vi "Data operation.vi"(8 "Output list":dbl[](array[numeric]), 9 "Operation":enum16{"Increase", "maintain", "Decrease"}(ring), 10 "Keithley Output Configure":T1={"Sample Count (10)"=10, "Timeout (10000 ms)"=10000, "Compliance  Level (0.1)"=0.1, "Output Level (0)"=0.0, "Source Mode  (0: Voltage)"=0, "Output sequence"=0, "Output list"=[]} {"Source Mode  (0: Voltage)" items=["Voltage", "Current"]; "Timeout (10000 ms)" format="%#.6g"}) -> (2 "Keithley Output Configure 2":T1={"Sample Count (10)"=10, "Timeout (10000 ms)"=10000, "Compliance  Level (0.1)"=0.1, "Output Level (0)"=0.0, "Source Mode  (0: Voltage)"=0, "Output sequence"=0, "Output list"=[]} {"Source Mode  (0: Voltage)" items=["Voltage", "Current"]; "Timeout (10000 ms)" format="%#.6g"})   [LabVIEW 2017]
uses:
  controls/Keithley input.ctl
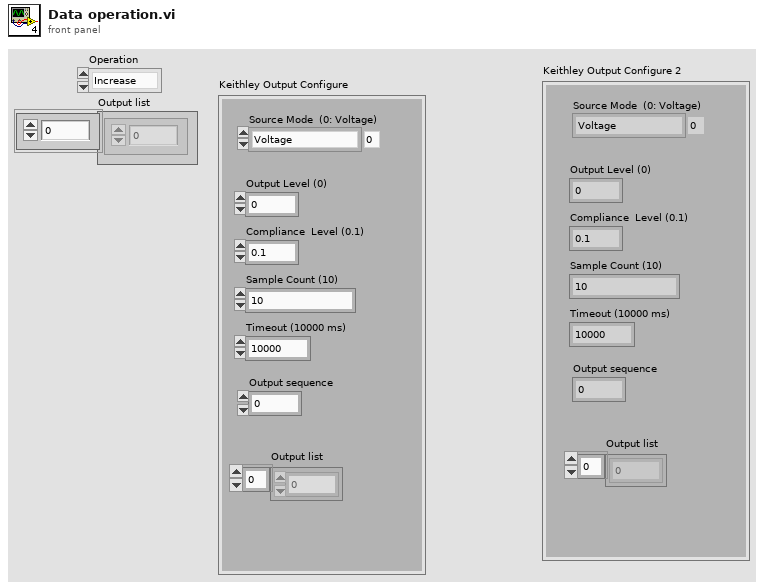
[diagram p1: front panel]
types:
  T1 = typedef "Keithley input.ctl" = cluster{"Sample Count (10)":i32, "Timeout (10000 ms)":i32, "Compliance  Level (0.1)":dbl, "Output Level (0)":dbl, "Source Mode  (0: Voltage)":u16, "Output sequence":i32, "Output list":dbl[]}
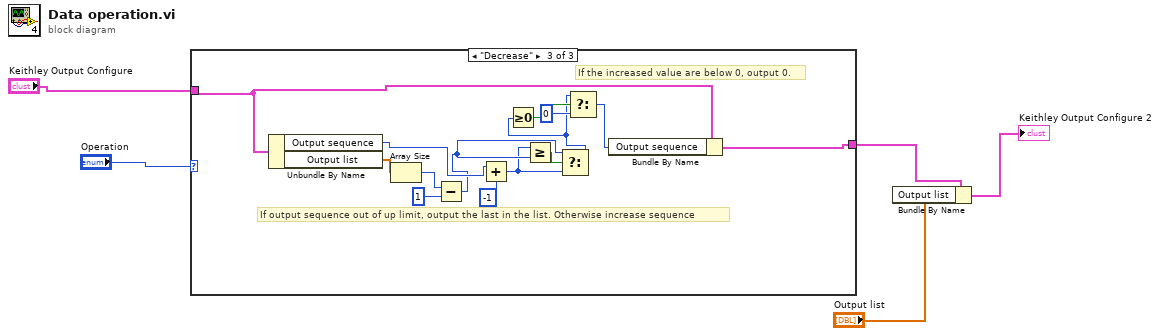
[diagram p0: block diagram]
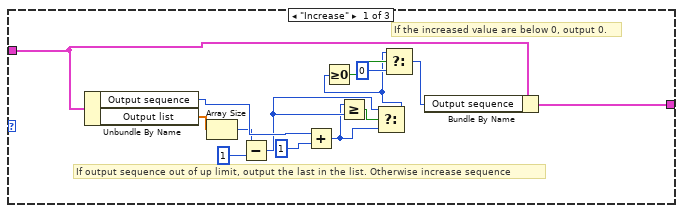
[diagram p2: hidden frame]
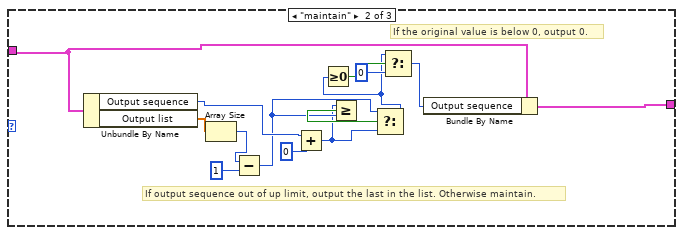
[diagram p3: hidden frame]
diagram:
  n1 = case shown="\"Decrease\"" "Operation" {
    tunnel: "Keithley Output Configure" -> [w10 w25 w38]
    tunnel: [w11 w24 w39] -> w3
    frame "Increase" {
      # "If the increased value are below 0, output 0."
      # "If output sequence out of up limit, output the last in the list. Otherwise increase sequence"
      n2 = Unbundle By Name(w10) -> ("Output sequence"=w16:i32, "Output list"=w19:dbl[])
      n3 = Array Size(array=w19) -> (size(s)=w8:i32)
      n4 = Subtract(x=w8, y=1) -> (x-y=w7:i32)
      n5 = Add(x=w16, y=1) -> (x+y=w6:i32)
      n6 = Greater Or Equal?(x=w6, y=w7) -> (x >= y?=w18:bool)
      n7 = Select(t=w7, s=w18, f=w6) -> (s? t:f=w12:i32)
      n8 = Greater Or Equal To 0?(x=w12) -> (x >= 0?=w15:bool)
      n9 = Select(t=w12, s=w15, f=0) -> (s? t:f=w13:i32)
      n10 = Bundle By Name(cluster=w10, "Output sequence"=w13) -> (w11:T1)
    }
    frame "maintain" {
      # "If the original value is below 0, output 0."
      # "If output sequence out of up limit, output the last in the list. Otherwise maintain."
      n11 = Unbundle By Name(w25) -> ("Output sequence"=w30:i32, "Output list"=w33:dbl[])
      n12 = Array Size(array=w33) -> (size(s)=w22:i32)
      n13 = Subtract(x=w22, y=1) -> (x-y=w21:i32)
      n14 = Add(x=w30, y=0) -> (x+y=w20:i32)
      n15 = Greater Or Equal?(x=w20, y=w21) -> (x >= y?=w32:bool)
      n16 = Select(t=w21, s=w32, f=w20) -> (s? t:f=w26:i32)
      n17 = Greater Or Equal To 0?(x=w26) -> (x >= 0?=w29:bool)
      n18 = Select(t=w26, s=w29, f=0) -> (s? t:f=w27:i32)
      n19 = Bundle By Name(cluster=w25, "Output sequence"=w27) -> (w24:T1)
    }
    frame "Decrease" {
      # "If the increased value are below 0, output 0."
      # "If output sequence out of up limit, output the last in the list. Otherwise increase sequence"
      n20 = Unbundle By Name(w38) -> ("Output sequence"=w44:i32, "Output list"=w47:dbl[])
      n21 = Array Size(array=w47) -> (size(s)=w36:i32)
      n22 = Subtract(x=w36, y=1) -> (x-y=w35:i32)
      n23 = Add(x=w44, y=-1) -> (x+y=w34:i32)
      n24 = Greater Or Equal?(x=w34, y=w35) -> (x >= y?=w46:bool)
      n25 = Select(t=w35, s=w46, f=w34) -> (s? t:f=w40:i32)
      n26 = Greater Or Equal To 0?(x=w40) -> (x >= 0?=w43:bool)
      n27 = Select(t=w40, s=w43, f=0) -> (s? t:f=w41:i32)
      n28 = Bundle By Name(cluster=w38, "Output sequence"=w41) -> (w39:T1)
    }
  }
  n29 = Bundle By Name(cluster=w3, "Output list"="Output list") -> (→"Keithley Output Configure 2":T1)
